vi "Decompose Cluster - String - Element Type.vi"() -> ()   [LabVIEW 2017, in "Composition.Tests.lvlib"]
uses:
  Composition.Tests.lvlib
  Composition/Composition.lvlib
  <vilib>/Utility/Data Type/NI_Data Type.lvlib
  <vilib>/Utility/Data Type/Type Definitions/Data Type.ctl
  <vilib>/addons/_JKI Toolkits/Caraya/classes/Assert/Assert.lvclass
  <vilib>/addons/_JKI Toolkits/Caraya/classes/Test/Test.lvclass
panel:
  out "error out":errorcluster
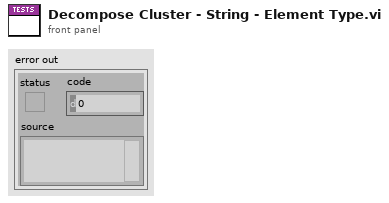
[diagram p1: front panel]
types:
  T1 = typedef "NI_Data Type.lvlib/Data Type.ctl" = enum8{"Invalid Type", "Void", "I8", "I16", "I32", "I64", "U8", "U16", "U32", "U64", "Single Float", "Double Float", "Extended Float", "Single Complex", "Double Complex", "Extended Complex", "Enum U8", "Enum U16", "Enum U32", "Enum U64", "Single Float With Unit", "Double Float With Unit", "Extended Float With Unit", "Single Complex with Unit", "Double Complex with Unit", "Extended Complex with Unit", "Boolean", "String", "Path", "Picture", "Tag", "Array", "Cluster", "Variant", "LV Variant", "Waveform", "Timestamp", "Digital Waveform", "Digital Data", "ExpressData", "Refnum", "External Data", "VI", "Poly VI", "LabVIEW Class Instance", "Fixed Point", "Set Collection", "Map Collection"}
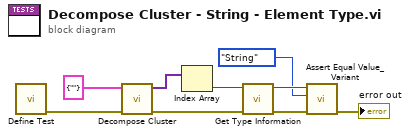
[diagram p0: block diagram]
diagram:
  n1 = call <vilib>:"Define Test.vi"() -> ("error out"=w1:errorcluster)  [unwired: 11 in]
  n2 = call "Decompose Cluster.vi"("error in (no error)"=w1, "Cluster"=cluster{string} {""}) -> ("error out"=w8:errorcluster, "Cluster Elements"=w6:variant[])  [unwired: 8 in]
  n3 = Index Array(array=w6) -> (element=w4:variant)  [unwired: 1 in]
  n4 = call <vilib>:"Get Type Information.vi"("error in (no error)"=w8, "variant"=w4) -> ("error out"=w7:errorcluster, "type"=w3:T1)  [unwired: 5 in, 3 out]
  n5 = call <vilib>:"Assert Equal Value_Variant.vi"("error in (no error)"=w7, "Y"=Data_Type."String" ("type"), "X"=w3) -> ("error out"=→"error out":errorcluster)  [unwired: 8 in]
